vi "GetScanCenterAndRadius.vi"(0 "System no.":i32=1 min=1 max=4 step=1, 1 "Gradient Scan Names":string[](array[string]), 2 "Scan Axes":string[](array[string]), 3 "Step Axes":string[](array[string]), 4 "Scan Routine Running?":bool[](array[boolean]), 5 "error in":errorcluster) -> (14 "Scan Axes Center":dbl[](array[numeric]), 15 "Step Axes Center":dbl[](array[numeric]), 16 "Current Radius":dbl[](array[numeric]), 19 "error out":errorcluster)   [LabVIEW 2020]
doc: "This VI queries gradient search routines radius and center position via FGC? and FRR? commands. If the routine is not running, POS? is used instead to query the position of the scan and step axis."
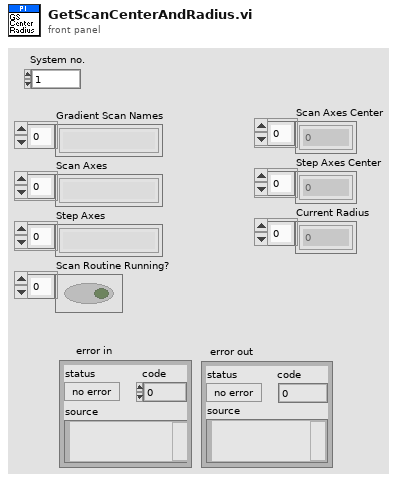
[diagram p1: front panel]
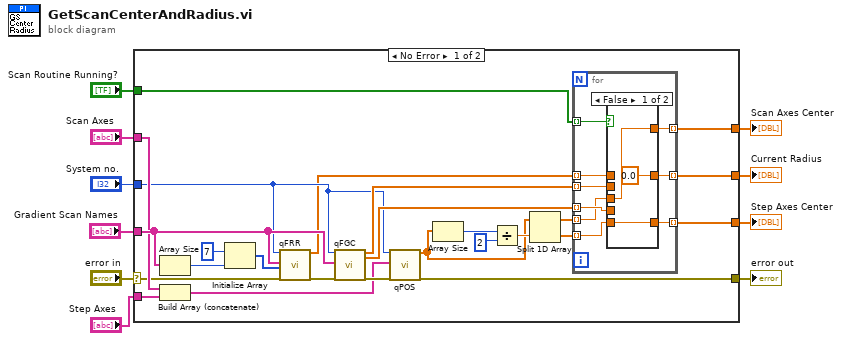
[diagram p0: block diagram]
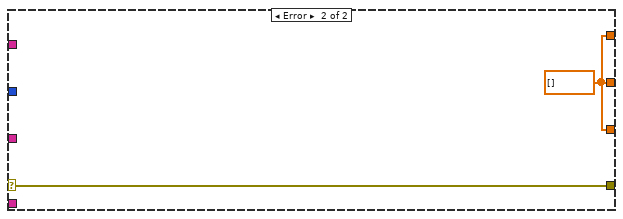
[diagram p3: hidden frame]
diagram:
  n1 = case shown="No Error" "error in" {
    selector: "error in" -> [w11 w52]
    tunnel: "Scan Routine Running?" -> [w28 _]
    tunnel: "Gradient Scan Names" -> [w27 _]
    tunnel: "Scan Axes" -> [w26 _]
    tunnel: "Step Axes" -> [w25 _]
    tunnel: "System no." -> [w23 _]
    tunnel: [w16 w51] -> w5
    tunnel: [w15 w51] -> w4
    tunnel: [w13 w51] -> w3
    tunnel: [w12 w52] -> w2
    frame No Error {
      n2 = Array Size(array=w27) -> (size(s)=w33:i32)
      n3 = Build Array (concatenate)(w26, w25) -> (w24:string[])
      n4 = Initialize Array(7 ("element"), w33) -> (w34:i32[])
      n5 = call "qFRR.vi"("System no."=w23, "Routinename"=w27, "ResultID"=w34, "error in"=w11) -> ("Value (num.)"=w14:dbl[], "error out"=w32:errorcluster)  [unwired: 2 in, 12 out]
      n6 = call "qFGC.vi"("System no."=w23, "Routine name"=w27, "error in"=w32) -> ("Scan axis center"=w30:dbl[], "Step axis center"=w29:dbl[], "error out"=w31:errorcluster)  [unwired: 1 in, 13 out]
      n7 = call "qPOS.vi"("System no."=w23, "Axes to query"=w24, "error in"=w31) -> ("Position"=w19:dbl[], "error out"=w12:errorcluster)  [unwired: 2 in, 13 out]
      n8 = Array Size(array=w19) -> (size(s)=w22:i32)
      n9 = Divide(x=w22, y=2) -> (x/y=w20:dbl)
      n10 = Split 1D Array(array=w19, index=w20) -> (first subarray=w18:dbl[], second subarray=w17:dbl[])
      n11 = for {
        tunnel: w28 -> [w44] mode=indexing
        tunnel: w18 -> [w39] mode=indexing
        tunnel: w17 -> [w38] mode=indexing
        tunnel: w30 -> [w43] mode=indexing
        tunnel: w29 -> [w42] mode=indexing
        tunnel: [w41] -> w16 mode=indexing
        tunnel: [w40] -> w15 mode=indexing
        tunnel: w14 -> [w37] mode=indexing
        tunnel: [w36] -> w13 mode=indexing
        n12 = case shown="False" w44 {
          tunnel: w43 -> [_ w50]
          tunnel: w42 -> [_ w49]
          tunnel: [w47 w50] -> w41
          tunnel: [w46 w49] -> w40
          tunnel: w39 -> [w47 _]
          tunnel: w38 -> [w46 _]
          tunnel: w37 -> [_ w48]
          tunnel: [0.0 ("Numeric") w48] -> w36
          frame False {
          }
          frame True {
          }
        }
      }
    }
    frame Error {
      w51 = dbl[] []
    }
  }
  "Scan Axes Center" <- w5
  "Step Axes Center" <- w4
  "Current Radius" <- w3
  "error out" <- w2
